vi "motor execute.vi"(7 "Command Motor":T2, 8 "error in":errorcluster, 9 "Value":variant, 10 "Param Cluster":T4={"Card"=1, "Num Dev"=1}, 11 "IOC":string(combo)) -> (0 "error out":errorcluster, 1 "Status":bool, 3 "Data Value Out":T3, 4 "PV Info":T1[](array[typedef]))   [LabVIEW 2022 SP3]
uses:
  pectus/control/epics value.ctl
  Program Files/National Instruments/LabVIEW 2023/user.lib/calab/PV Info.ctl
  Program Files/National Instruments/LabVIEW 2023/user.lib/calab/CaLab.lvlib
  578652f1-3f65-4d0d-86e6-664bc2074718.vi
  ccc3fe50-a785-4602-93ae-d66848f1026a.vi
  6c3fd1b2-ce51-4043-a194-d6392e3bfd3f.vi
  8f5b5cbe-28fe-4c2f-82ec-c9ca473c1fdb.vi
  pectus/control/Param Epics Cluster.ctl
  pectus/control/cast fe motor.ctl
panel:
  in  "Value Test":dbl
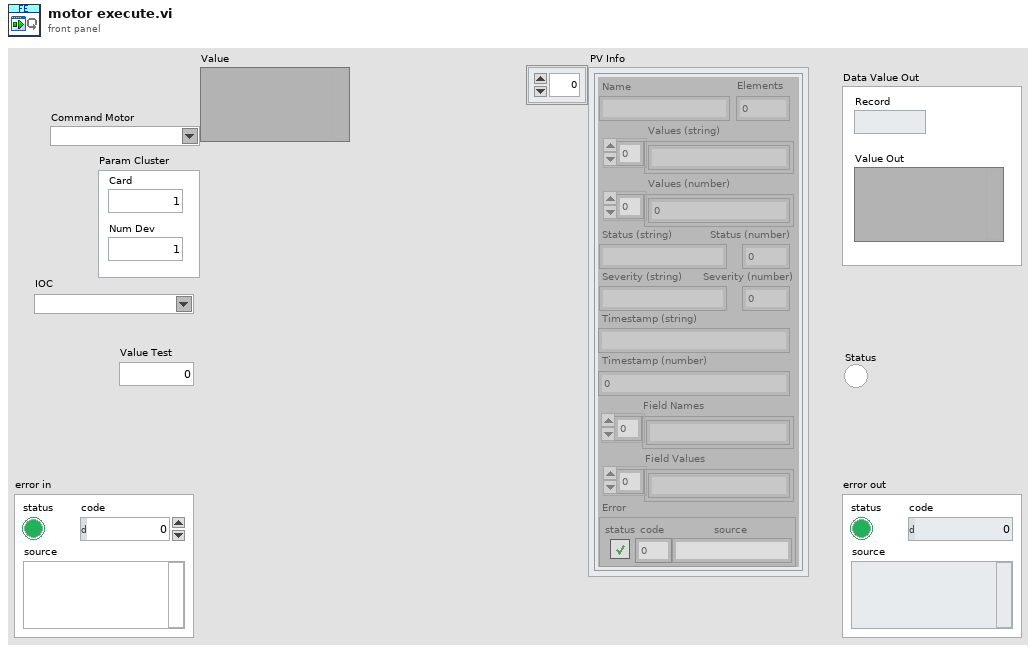
[diagram p1: front panel]
types:
  T1 = typedef "CaLab.lvlib/PV Info.ctl" = cluster{"Name":string, "Elements":i32, "Values (string)":string[], "Values (number)":dbl[], "Status (string)":string, "Status (number)":i16, "Severity (string)":string, "Severity (number)":i16, "Timestamp (string)":string, "Timestamp (number)":i32, "Field Names":string[], "Field Values":string[], "Error":errorcluster}
  T2 = typedef "cast fe motor.ctl" = string
  T3 = typedef "epics value.ctl" = cluster{"Record":string, "Value Out":variant}
  T4 = typedef "Param Epics Cluster.ctl" = cluster{"Card":u16, "Num Dev":u16}
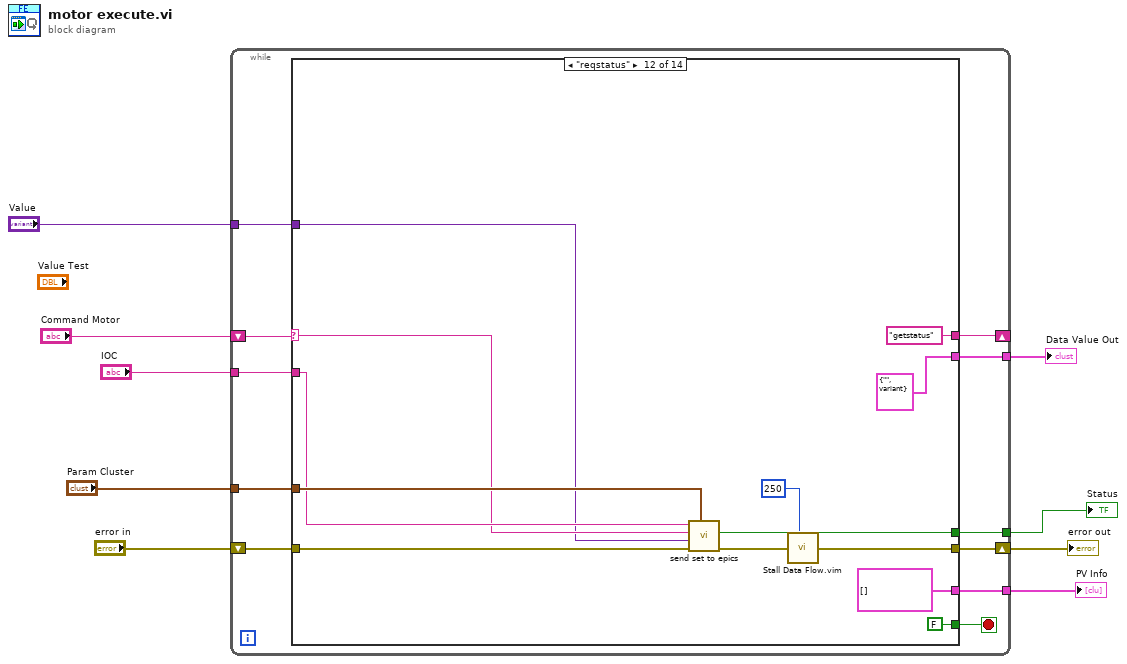
[diagram p0: block diagram]
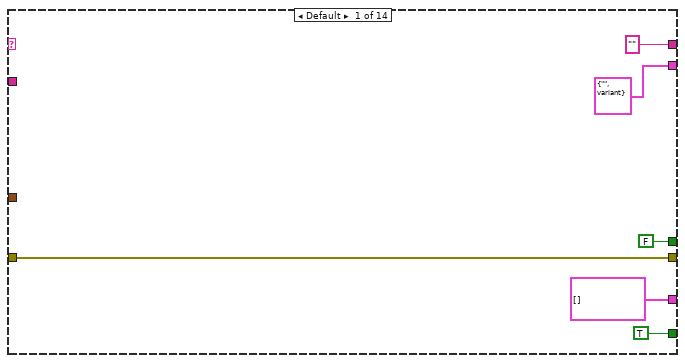
[diagram p2: hidden frame]
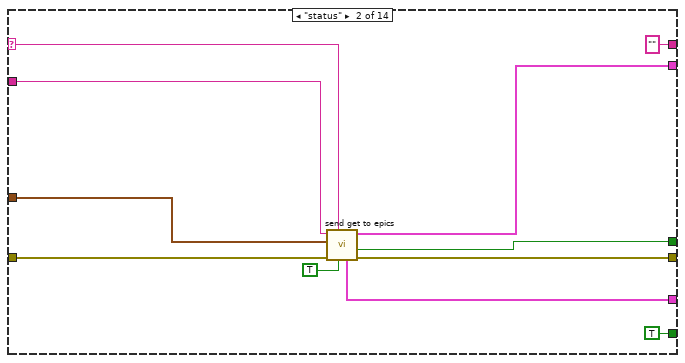
[diagram p3: hidden frame]
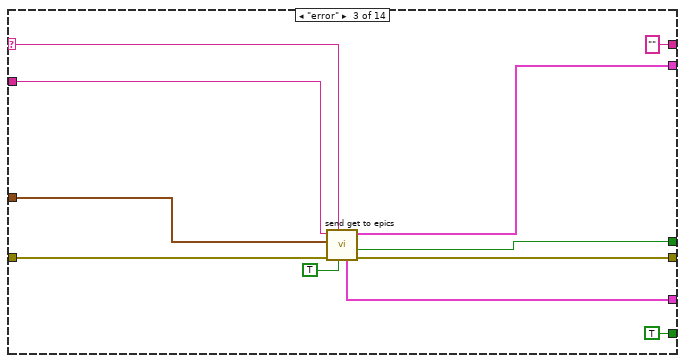
[diagram p4: hidden frame]
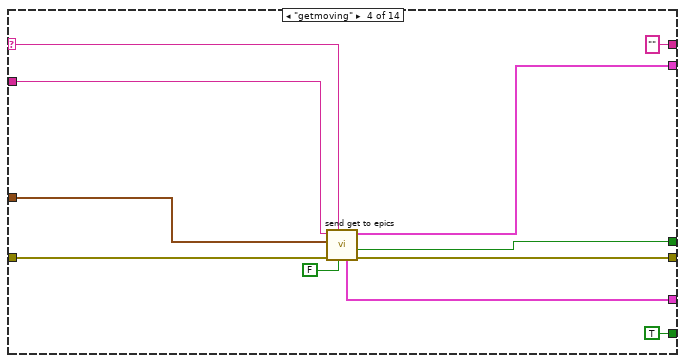
[diagram p5: hidden frame]
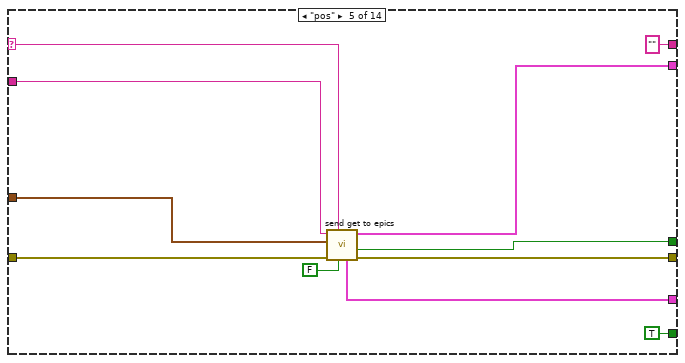
[diagram p6: hidden frame]
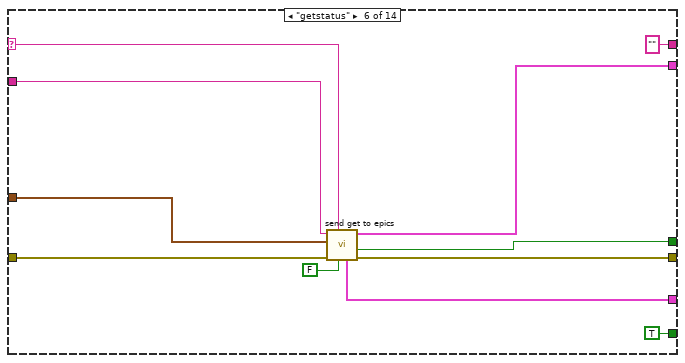
[diagram p7: hidden frame]
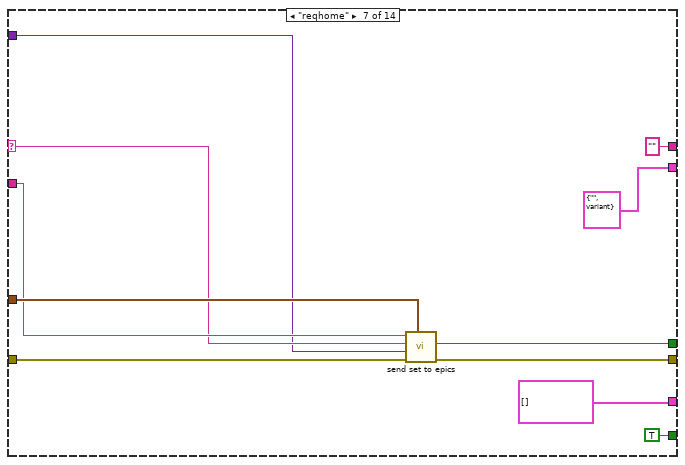
[diagram p8: hidden frame]
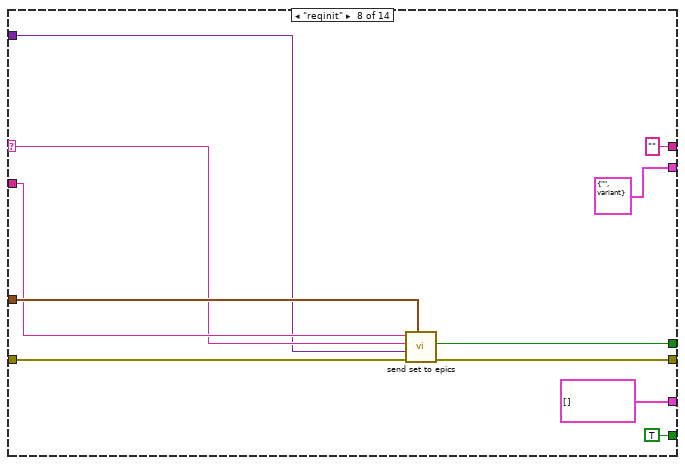
[diagram p9: hidden frame]
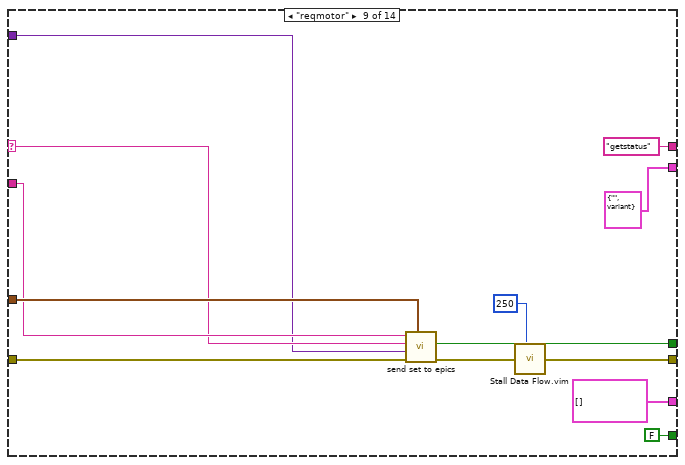
[diagram p10: hidden frame]
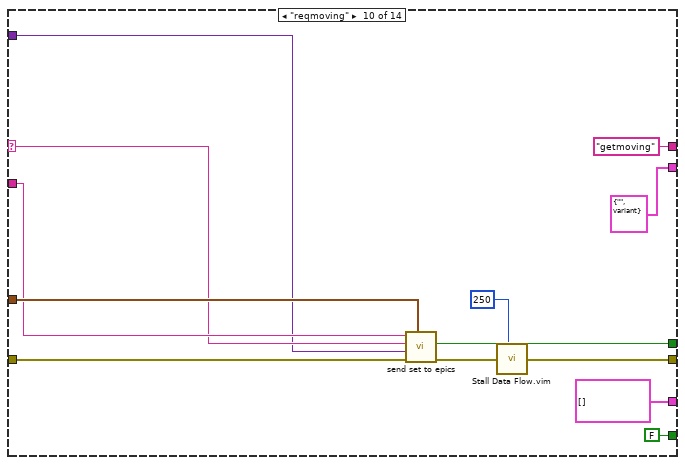
[diagram p11: hidden frame]
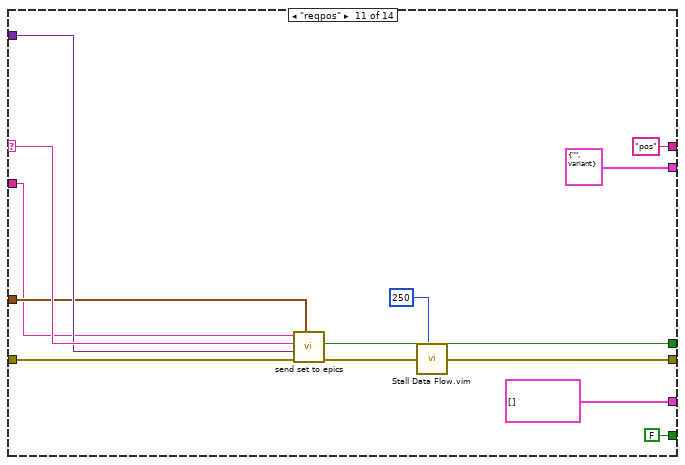
[diagram p12: hidden frame]
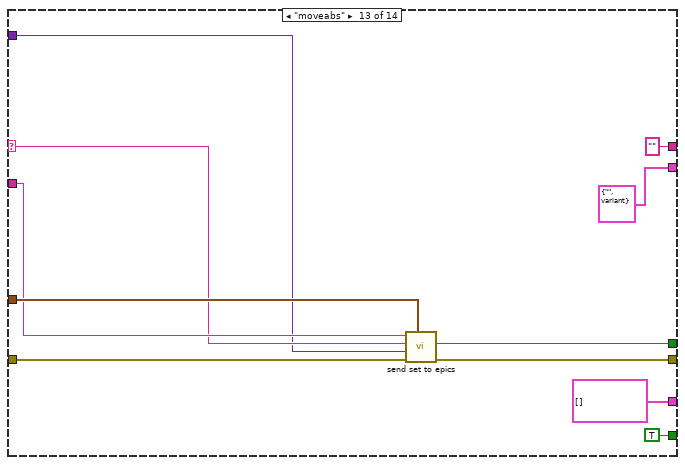
[diagram p13: hidden frame]
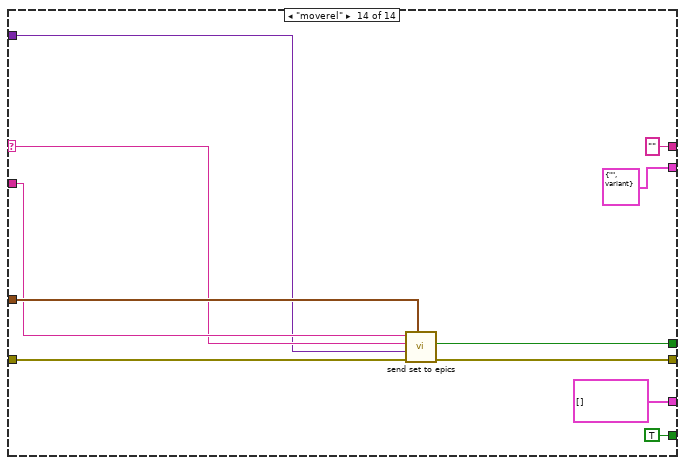
[diagram p14: hidden frame]
diagram:
  n1 = while {
    tunnel: [w17] -> w6
    tunnel: [w16] -> w5
    tunnel: "Param Cluster" -> [w14]
    tunnel: "Value" -> [w13]
    tunnel: [w12] -> w1
    shift-right: [w20] -> w9
    shift-left: "error in" -> [w19]
    tunnel: "IOC" -> [w18]
    shift-right: [w10] -> _
    shift-left: "Command Motor" -> [w15]
    stop <- w11 stop-if-true
    n2 = case shown="\"reqstatus\"" w15 {
      selector: w15 -> [_ w30 w41 w52 w63 w74 w87 w98 w112 w125 w141 w151 w161 w172]
      tunnel: [w26 w36 w47 w58 w69 w80 w91 w102 w104 w117 w130 w143 w165 w176] -> w20
      tunnel: w19 -> [w26 w37 w48 w59 w70 w81 w92 w103 w116 w129 w142 w155 w166 w177]
      tunnel: w18 -> [_ w31 w42 w53 w64 w75 w88 w99 w113 w126 w138 w152 w162 w173]
      tunnel: [FALSE ("Status") w35 w46 w57 w68 w79 w90 w101 w115 w128 w137 w154 w164 w175] -> w17
      tunnel: [T3 {"Record"="", "Value Out"=variant} ("Data Value Out") w34 w45 w56 w67 w78 T3 {"Record"="", "Value Out"=variant} ("Data Value Out") T3 {"Record"="", "Value Out"=variant} ("Data Value Out") T3 {"Record"="", "Value Out"=variant} ("Data Value Out") T3 {"Record"="", "Value Out"=variant} ("Data Value Out") T3 {"Record"="", "Value Out"=variant} ("Data Value Out") T3 {"Record"="", "Value Out"=variant} ("Data Value Out") T3 {"Record"="", "Value Out"=variant} ("Data Value Out") T3 {"Record"="", "Value Out"=variant} ("Data Value Out")] -> w16
      tunnel: w14 -> [_ w32 w43 w54 w65 w76 w89 w100 w114 w127 w139 w153 w163 w174]
      tunnel: w13 -> [_ _ _ _ _ _ w86 w97 w111 w124 w140 w150 w160 w171]
      tunnel: [T1[] [] ("PV Info") w29 w40 w51 w62 w73 T1[] [] ("PV Info") T1[] [] ("PV Info") T1[] [] ("PV Info") T1[] [] ("PV Info") T1[] [] ("PV Info") T1[] [] ("PV Info") T1[] [] ("PV Info") T1[] [] ("PV Info")] -> w12
      tunnel: [TRUE TRUE TRUE TRUE TRUE TRUE TRUE TRUE FALSE FALSE FALSE FALSE TRUE TRUE] -> w11
      tunnel: ["" ("Value Out - String") "" ("Value Out - String") "" ("Value Out - String") "" ("Value Out - String") "" ("Value Out - String") "" ("Value Out - String") "" ("Value Out - String") "" ("Value Out - String") "getstatus" ("Value Out - String") "getmoving" ("Value Out - String") "pos" ("Value Out - String") "getstatus" ("Value Out - String") "" ("Value Out - String") "" ("Value Out - String")] -> w10
      frame Default {
      }
      frame "status" {
        n3 = call "send get to epics.vi"("to PROC?"=TRUE, "Command"=w30, "error in"=w37, "Param Cluster"=w32, "IOC"=w31) -> ("error out"=w36:errorcluster, "Status"=w35:bool, "Data Value Out"=w34:T3, "PV Info"=w29:T1[])  [unwired: 3 in]
      }
      frame "error" {
        n4 = call "send get to epics.vi"("to PROC?"=TRUE, "Command"=w41, "error in"=w48, "Param Cluster"=w43, "IOC"=w42) -> ("error out"=w47:errorcluster, "Status"=w46:bool, "Data Value Out"=w45:T3, "PV Info"=w40:T1[])  [unwired: 3 in]
      }
      frame "getmoving" {
        n5 = call "send get to epics.vi"("to PROC?"=FALSE, "Command"=w52, "error in"=w59, "Param Cluster"=w54, "IOC"=w53) -> ("error out"=w58:errorcluster, "Status"=w57:bool, "Data Value Out"=w56:T3, "PV Info"=w51:T1[])  [unwired: 3 in]
      }
      frame "pos" {
        n6 = call "send get to epics.vi"("to PROC?"=FALSE, "Command"=w63, "error in"=w70, "Param Cluster"=w65, "IOC"=w64) -> ("error out"=w69:errorcluster, "Status"=w68:bool, "Data Value Out"=w67:T3, "PV Info"=w62:T1[])  [unwired: 3 in]
      }
      frame "getstatus" {
        n7 = call "send get to epics.vi"("to PROC?"=FALSE, "Command"=w74, "error in"=w81, "Param Cluster"=w76, "IOC"=w75) -> ("error out"=w80:errorcluster, "Status"=w79:bool, "Data Value Out"=w78:T3, "PV Info"=w73:T1[])  [unwired: 3 in]
      }
      frame "reqhome" {
        n8 = call "send set to epics.vi"("Param Cluster"=w89, "error in"=w92, "Value"=w86, "select"=w87, "IOC Selected"=w88) -> ("error out"=w91:errorcluster, "Status"=w90:bool)  [unwired: 5 in]
      }
      frame "reqinit" {
        n9 = call "send set to epics.vi"("Param Cluster"=w100, "error in"=w103, "Value"=w97, "select"=w98, "IOC Selected"=w99) -> ("error out"=w102:errorcluster, "Status"=w101:bool)  [unwired: 5 in]
      }
      frame "reqmotor" {
        n10 = call "send set to epics.vi"("Param Cluster"=w114, "error in"=w116, "Value"=w111, "select"=w112, "IOC Selected"=w113) -> ("error out"=w105:errorcluster, "Status"=w115:bool)  [unwired: 5 in]
        n11 = call "Stall Data Flow.vim"("value in"=w105, "milliseconds to wait"=u32 250) -> ("value out"=w104:errorcluster)  [unwired: 1 out]
      }
      frame "reqmoving" {
        n12 = call "send set to epics.vi"("Param Cluster"=w127, "error in"=w129, "Value"=w124, "select"=w125, "IOC Selected"=w126) -> ("error out"=w118:errorcluster, "Status"=w128:bool)  [unwired: 5 in]
        n13 = call "Stall Data Flow.vim"("value in"=w118, "milliseconds to wait"=u32 250) -> ("value out"=w117:errorcluster)  [unwired: 1 out]
      }
      frame "reqpos" {
        n14 = call "send set to epics.vi"("Param Cluster"=w139, "error in"=w142, "Value"=w140, "select"=w141, "IOC Selected"=w138) -> ("error out"=w131:errorcluster, "Status"=w137:bool)  [unwired: 5 in]
        n15 = call "Stall Data Flow.vim"("value in"=w131, "milliseconds to wait"=u32 250) -> ("value out"=w130:errorcluster)  [unwired: 1 out]
      }
      frame "reqstatus" {
        n16 = call "send set to epics.vi"("Param Cluster"=w153, "error in"=w155, "Value"=w150, "select"=w151, "IOC Selected"=w152) -> ("error out"=w144:errorcluster, "Status"=w154:bool)  [unwired: 5 in]
        n17 = call "Stall Data Flow.vim"("value in"=w144, "milliseconds to wait"=u32 250) -> ("value out"=w143:errorcluster)  [unwired: 1 out]
      }
      frame "moveabs" {
        n18 = call "send set to epics.vi"("Param Cluster"=w163, "error in"=w166, "Value"=w160, "select"=w161, "IOC Selected"=w162) -> ("error out"=w165:errorcluster, "Status"=w164:bool)  [unwired: 5 in]
      }
      frame "moverel" {
        n19 = call "send set to epics.vi"("Param Cluster"=w174, "error in"=w177, "Value"=w171, "select"=w172, "IOC Selected"=w173) -> ("error out"=w176:errorcluster, "Status"=w175:bool)  [unwired: 5 in]
      }
    }
  }
  "error out" <- w9
  "Status" <- w6
  "Data Value Out" <- w5
  "PV Info" <- w1
